vi "standard deviations from power spectrum array.vi"(11 "pwer spectran":cluster{"f0":dbl, "df":dbl, "magnitude":dbl[]}[](array[cluster])) -> (3 "standard deviations":dbl[](array[numeric]))   [LabVIEW 2020]
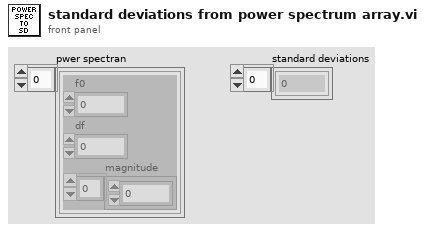
[diagram p1: front panel]
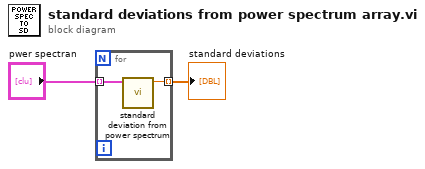
[diagram p0: block diagram]
diagram:
  n1 = for {
    tunnel: "pwer spectran" -> [w4] mode=indexing
    tunnel: [w3] -> w2 mode=indexing
    n2 = call "standard deviation from power spectrum.vi"("Power Spectrum"=w4) -> ("Numeric"=w3:dbl)  [unwired: 10 in]
  }
  "standard deviations" <- w2
